vi "PlannedPath_set.vi"(8 "error in (no error)":errorcluster, 10 "PlannedPath":cluster{"X position":dbl, "Y position":dbl}[](array[cluster])) -> (0 "error out":errorcluster)   [LabVIEW 2009, in "NetworkVarTarget.lvlib"]
uses:
  NetworkVarTarget.lvlib
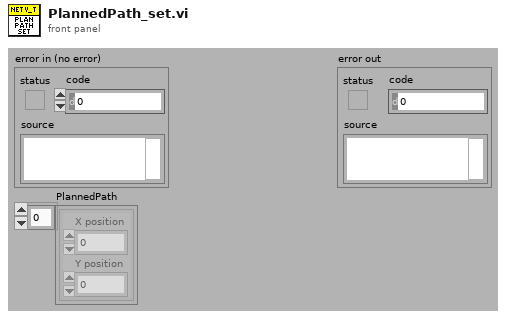
[diagram p1: front panel]
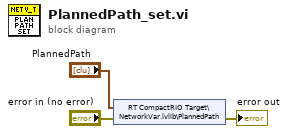
[diagram p0: block diagram]
diagram:
  n1 = shared-variable "RT CompactRIO Target\\NetworkVar.lvlib\\PlannedPath"("PlannedPath", error in="error in (no error)") -> (error out=→"error out":errorcluster)
